vi "SubVI_Histogram.vi"(7 "Image Register Name":string="untitled", 8 "Error in":errorcluster, 10 "ROI Descriptor":T1 {"Contours"."Type" items=["No Selection", "Point", "Line", "Rectangle", "Oval", "Polygon", "Freehand Region", "Annulus", "Unused2", "Unused3", "Broken Line", "Freehand Line", "Rotated Rectangle"]}, 11 "Image Sorce In":T2) -> (0 "Error out":errorcluster, 2 "Mean Value":i32, 3 "Image Sorce Out":T2)   [LabVIEW 2013]
uses:
  <vilib>/vision/Image Controls.llb/IMAQ Image.ctl
  <vilib>/vision/NI_Vision_Development_Module.lvlib
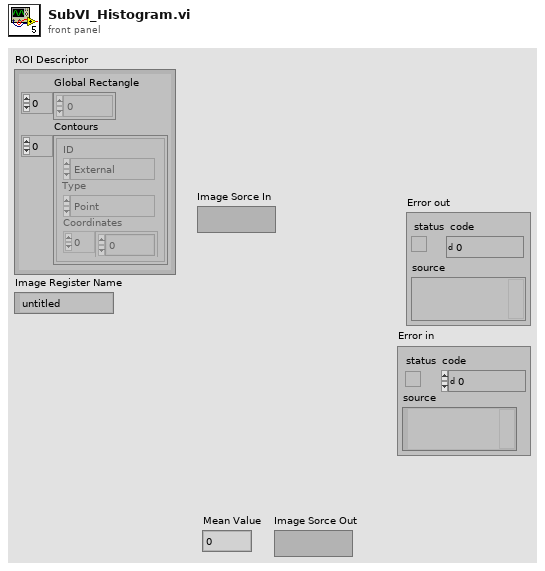
[diagram p1: front panel]
types:
  T1 = typedef "ROI Descriptor" = cluster{"Global Rectangle":i32[], "Contours":cluster{"ID":enum32{"External", "Internal"}, "Type":u32, "Coordinates":i32[]}[]}
  T2 = typedef "IMAQ Image.ctl" = refnum<image>
  T3 = typedef "Image Type" = u32
  T4 = cluster{"histogram":u32[], "Minimal Value":sgl, "Maximal Value":sgl, "Starting Value":sgl, "Interval Width":sgl, "Mean Value":sgl, "Standard  Variation":sgl, "Area (pixels)":i32}
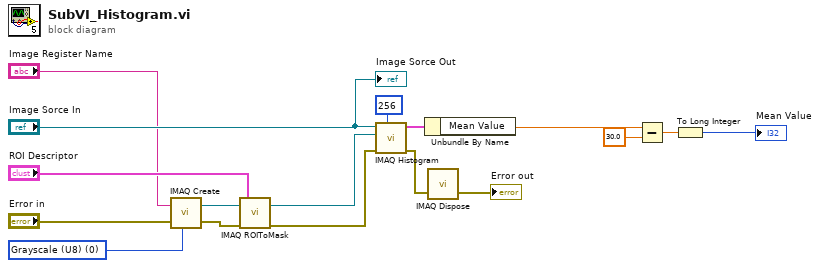
[diagram p0: block diagram]
diagram:
  w7 = T3 0 items=["Grayscale (U8)", "Grayscale (I16)", "Grayscale (SGL)", "Complex (CSG)", "RGB (U32)", "HSL (U32)", "RGB (U64)", "Grayscale (U16)"] ("Image Type")
  n1 = call "IMAQ Create"("Image Name"="Image Register Name", "Image Type"=w7, "error in (no error)"="Error in") -> ("New Image"=w8:T2, "error out"=w3:errorcluster)  [unwired: 1 in, 1 out]
  n2 = call "IMAQ ROIToMask"("error in (no error)"=w3, "ROI Descriptor"="ROI Descriptor", "Image"=w8) -> ("error out"=w5:errorcluster, "Image Out"=w6:T2)  [unwired: 2 in, 2 out]
  n3 = call "IMAQ Histogram"("Number of Classes"=256, "error in (no error)"=w5, "Image Mask"=w6, "Image"="Image Sorce In") -> ("error out"=w15:errorcluster, "Histogram Report"=w16:T4)  [unwired: 1 in, 5 out]
  n4 = Unbundle By Name(w16) -> ("Mean Value"=w11:sgl)
  n5 = call "IMAQ Dispose"("error in (no error)"=w15) -> ("error out"=→"Error out":errorcluster)  [unwired: 5 in]
  n6 = Subtract(x=w11, y=sgl 30.0) -> (x-y=w10:sgl)
  n7 = To Long Integer(number=w10) -> (32bit integer=→"Mean Value":i32)
  "Image Sorce Out" <- "Image Sorce In"
